vi "Time Difference.vi"(7 "Time1":string="09-03-2021 10:23:34", 9 "Time2":string="09-03-2021 11:24:34") -> (0 "error out":errorcluster, 2 "Time Stamp Indicator - Long 6":timestamp format="%<%H:%M:%S>T")   [LabVIEW 2017]
doc: "AMEE"
panel:
  out "Elapsed Time":string
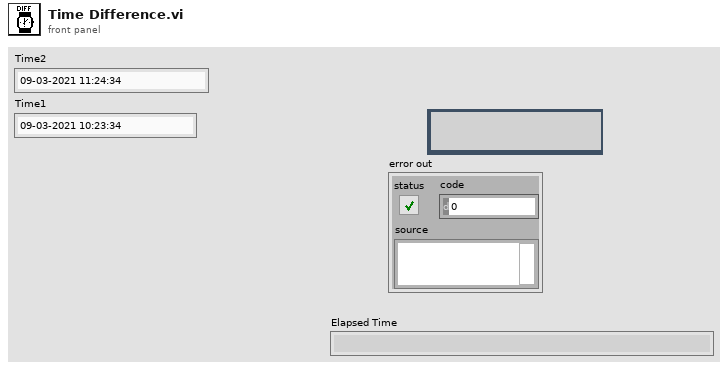
[diagram p1: front panel]
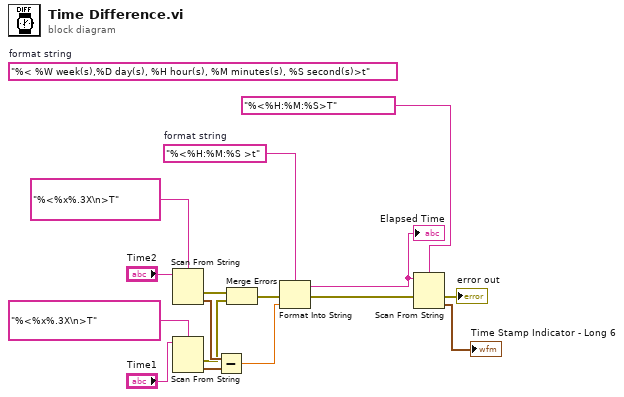
[diagram p0: block diagram]
diagram:
  (unwired) "%< %W week(s),%D day(s), %H hour(s), %M minutes(s), %S second(s)>t"  # format string
  w16 = "%<%H:%M:%S >t"  # format string
  n1 = Scan From String(format string="%<%x%.3X\n>T", input string="Time2") -> (error out=w5:errorcluster, output 1=w10:timestamp)  [unwired: 3 in, 2 out]
  n2 = Scan From String(format string="%<%x%.3X\n>T", input string="Time1") -> (error out=w4:errorcluster, output 1=w7:timestamp)  [unwired: 3 in, 2 out]
  n3 = Subtract(x=w10, y=w7) -> (x-y=w15:dbl)
  n4 = Merge Errors(w5, w4) -> (w3:errorcluster)
  n5 = Format Into String "Format Into String"(format string=w16, error in=w3, w15) -> (resulting string=w14:string, error out=w2:errorcluster)  [unwired: 1 in]
  "Elapsed Time" <- w14
  n6 = Scan From String(format string="%<%H:%M:%S>T", input string=w14, error in=w2) -> (error out=→"error out":errorcluster, output 1=→"Time Stamp Indicator - Long 6":timestamp)  [unwired: 2 in, 2 out]
